vi "Get_SENSOR.vi"(11 "CODE_MAIN":string) -> (3 "CODE_SENSOR":string)   [LabVIEW 2020]
uses:
  Global_Variable/Global.vi
panel:
  out "error out":errorcluster
  in  "error in (no error)":errorcluster
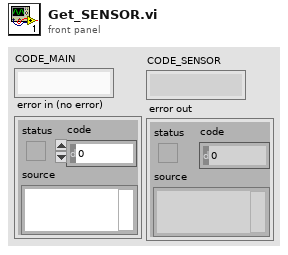
[diagram p1: front panel]
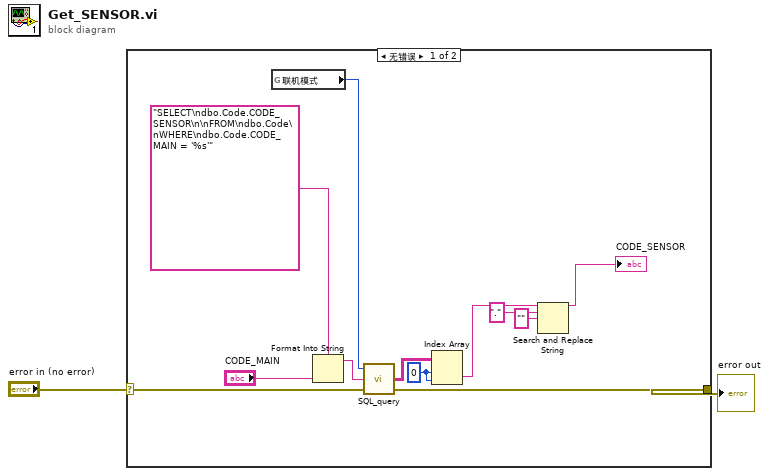
[diagram p0: block diagram]
diagram:
  n1 = case shown="无错误" "error in (no error)" {
    selector: "error in (no error)" -> [w10 w15]
    tunnel: [w9 w15] -> w1
    frame No Error {
      w7 = 0 ("索引 (行)")
      n2 = global read "Global.vi" "联机模式"() -> (w12:enum16{"单机", "追溯"})
      n3 = Format Into String(format string="SELECT\ndbo.Code.CODE_SENSOR\n\nFROM\ndbo.Code\nWHERE\ndbo.Code.CODE_MAIN = '%s'" ("格式字符串"), "CODE_MAIN") -> (resulting string=w11:string)  [unwired: 2 in, 1 out]
      n4 = call "SQL_query.vi"("error in (no error)"=w10, "SQL query"=w11, "联机模式"=w12) -> ("error out"=w9:errorcluster, "data"=w8:string[][])  [unwired: 1 in]
      n5 = Index Array(array=w8, index (row)=w7, index (col)=w7) -> (element=w6:string)
      n6 = Search and Replace String(input string=w6, search string="." ("搜索字符串"), replace string="" ("替换字符串(\"\")")) -> (result string=→"CODE_SENSOR":string)  [unwired: 5 in, 3 out]
    }
    frame Error {
    }
  }
  "error out" <- w1
